vi "Compress.vi"(4 "No of threads":i32, 6 "Compression Level":i32=3, 8 "error in (no error)":errorcluster, 10 "data in":string) -> (0 "error out":errorcluster, 2 "compressed data":string)   [LabVIEW 2020, in "lvzstd.lvlib"]
uses:
  lvzstd.lvlib
  Private/Path FGV.vi
  <vilib>/Utility/error.llb/Error Cluster From Error Code.vi
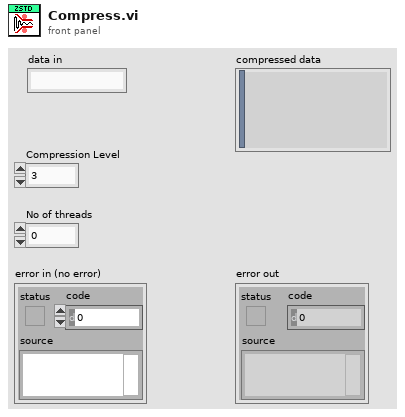
[diagram p1: front panel]
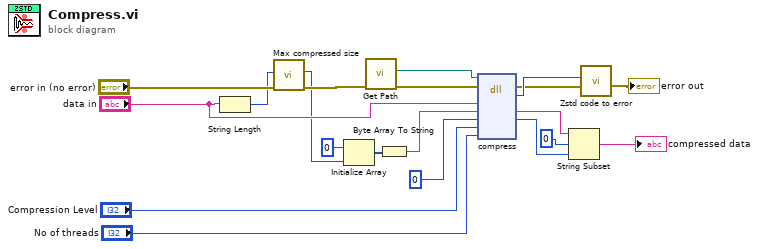
[diagram p0: block diagram]
diagram:
  n1 = String Length(string="data in") -> (length=w2:i32)
  n2 = call "Max compressed size.vi"("error in (no error)"="error in (no error)", "source size (bytes)"=w2) -> ("error out"=w3:errorcluster, "maximum compressed size (bytes)"=w1:i32)  [unwired: 8 in]
  n3 = Initialize Array(u8 0, w1) -> (w17:u8[])
  n4 = call "Get Path.vi"("error in (no error)"=w3) -> ("error out (no error)"=w6:errorcluster, "Library Path"=w5:path)  [unwired: 9 in]
  n5 = Byte Array To String(unsigned byte array=w17) -> (string=w16:string)
  n6 = dll-call lib="?" fn="compress"(path in=w5, error in=w6, "srcHandle"="data in", "dstHandle"=w16, "compressedSize"=0, "cLevel"="Compression Level", "noThreads"="No of threads") -> (error out=w8:errorcluster, "return type"=w12:i32, "dstHandle"=w11:string, "compressedSize"=w15:i32)  [unwired: 4 in, 1 out]
  n7 = String Subset(string=w11, offset (0)=0, length (rest)=w15) -> (substring=→"compressed data":string)
  n8 = call "Zstd code to error.vi"("error in"=w8, "Error code"=w12) -> ("error in (no error)"=→"error out":errorcluster)  [unwired: 9 in]
